vi "thermocouple_run.vi"(8 "error in (no error)":errorcluster, 9 "volume rise per 1C":dbl, 10 "max volume":dbl, 11 "Refnum in":refnum<k21>) -> (0 "error out":errorcluster, 1 "volume":dbl, 3 "task out":refnum<k21>)   [LabVIEW 2022 SP3]
uses:
  <vilib>/DAQmx/read.llb/DAQmx Read (Analog DBL 1Chan 1Samp).vi
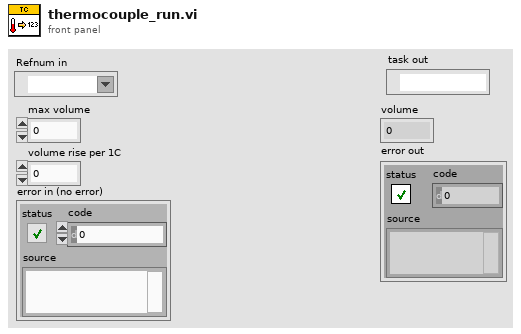
[diagram p1: front panel]
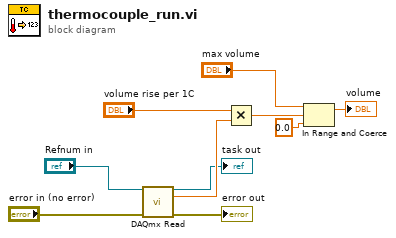
[diagram p0: block diagram]
diagram:
  n1 = call-poly <vilib>:"DAQmx Read.vi"("task/channels in"="Refnum in", "error in"="error in (no error)") -> ("task out"=→"task out":refnum<k21>, "data"=w4:dbl, "error out"=→"error out":errorcluster)  [unwired: 11 in]
  n2 = Multiply(x="volume rise per 1C", y=w4) -> (x*y=w7:dbl)
  n3 = In Range and Coerce(upper limit="max volume", x=w7, lower limit=0.0) -> (coerced(x)=→"volume":dbl)  [unwired: 1 out]
